vi "SNAP_PHOTO.vi"(10 "Image":T1, 11 "Boolean":bool) -> (3 "Numeric 2":i32)   [LabVIEW 2015]
uses:
  <vilib>/vision/Image Controls.llb/IMAQ Image.ctl
panel:
  in  "Boolean 3":bool
  in  "Numeric":i32
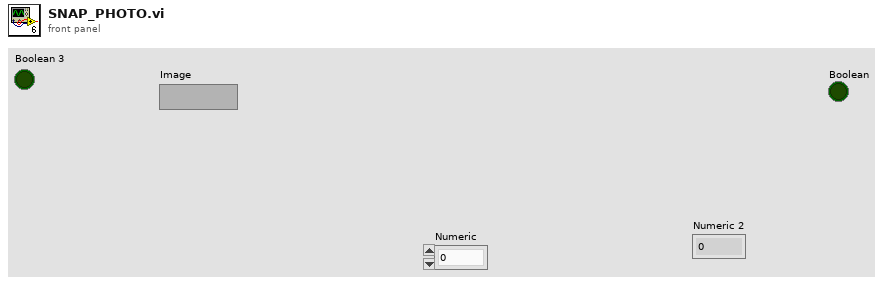
[diagram p1: front panel]
types:
  T1 = typedef "IMAQ Image.ctl" = refnum<image>
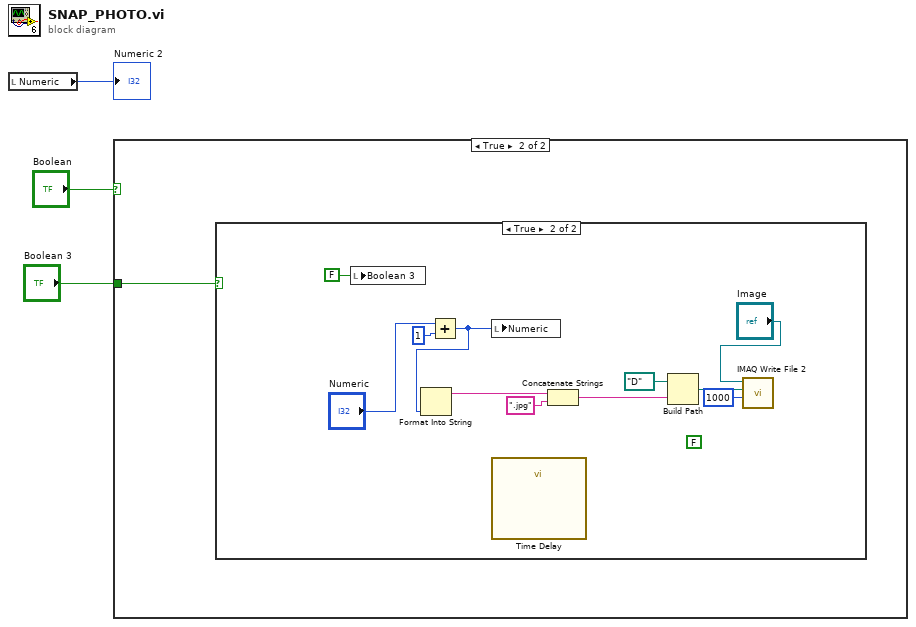
[diagram p0: block diagram]
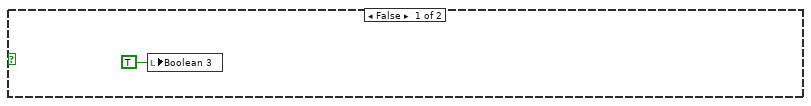
[diagram p2: hidden frame]
diagram:
  n1 = local read "Numeric"() -> (→"Numeric 2":i32)
  n2 = case shown="True" "Boolean" {
    tunnel: "Boolean 3" -> [_ w5]
    frame False {
      n3 = local write "Boolean 3"(TRUE) -> ()
    }
    frame True {
      n4 = case shown="True" w5 {
        frame False {
        }
        frame True {
          (unwired) FALSE ("Compress? (N)")
          n5 = local write "Boolean 3"(FALSE) -> ()
          n6 = Add(x="Numeric", y=1) -> (x+y=w7:i32)
          n7 = Format Into String(w7) -> (resulting string=w14:string)  [unwired: 3 in, 1 out]
          n8 = local write "Numeric"(w7) -> ()
          n9 = call "Time Delay"() -> ()  [unwired: 11 in, 1 out]
          n10 = Concatenate Strings(w14, ".jpg" ("string")) -> (w12:string)
          n11 = Build Path(base path=path "D:/", name or relative path=w12) -> (appended path=w11:path)
          n12 = call-poly "IMAQ Write File 2"("Image Quality"=u32 1000, "File Path"=w11, "Image"="Image") -> ()  [unwired: 7 in, 2 out]
        }
      }
    }
  }
